vi "User Event Print.vi"(7 "Options":T1, 8 "error in (no error)":errorcluster, 9 "add EOL? (T)":bool=TRUE, 11 "String to Print":string) -> (0 "error out":errorcluster, 3 "Print":refnum<user-event>)   [LabVIEW 2018]
uses:
  Print Options.ctl
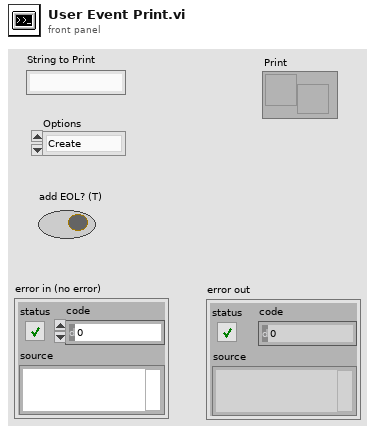
[diagram p1: front panel]
types:
  T1 = typedef "Print Options.ctl" = enum16{"Create", "Get Reference", "Print", "Print Header", "Close"}
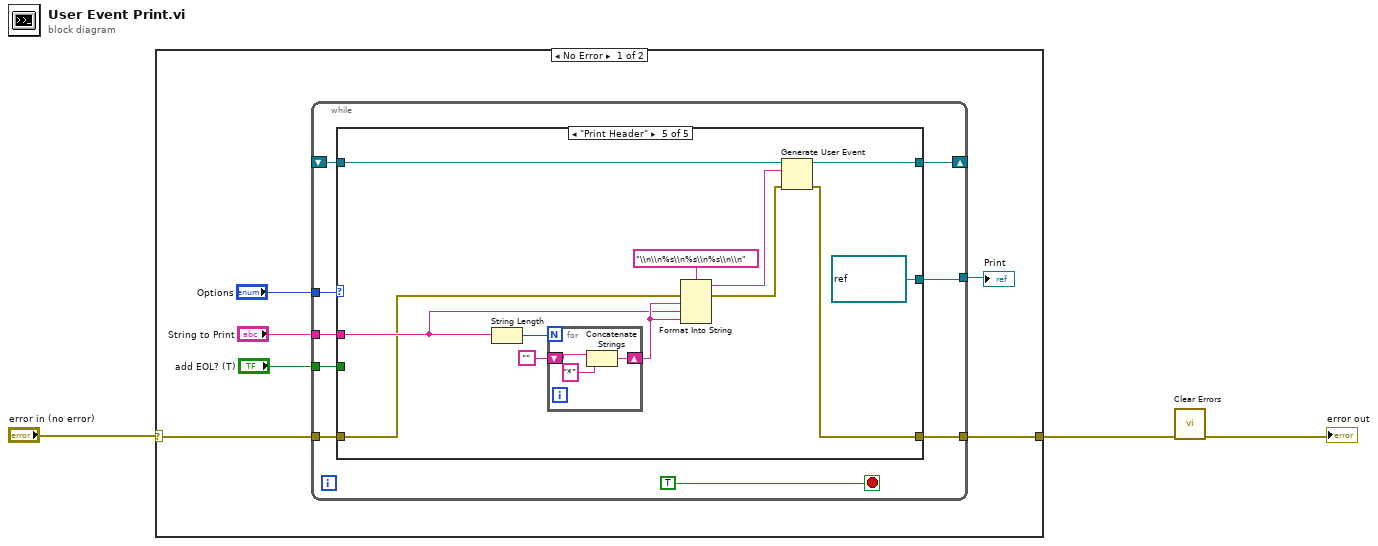
[diagram p0: block diagram]
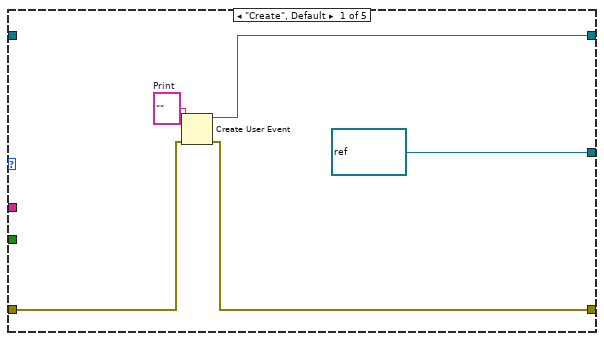
[diagram p2: hidden frame]
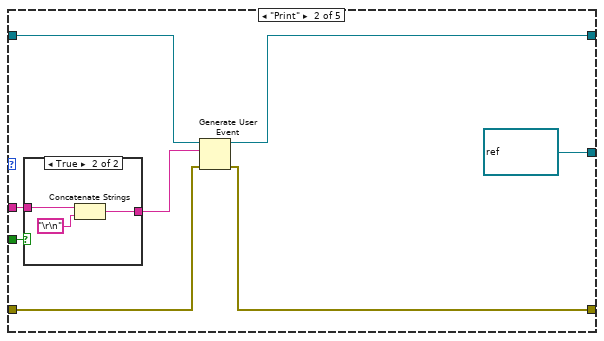
[diagram p3: hidden frame]
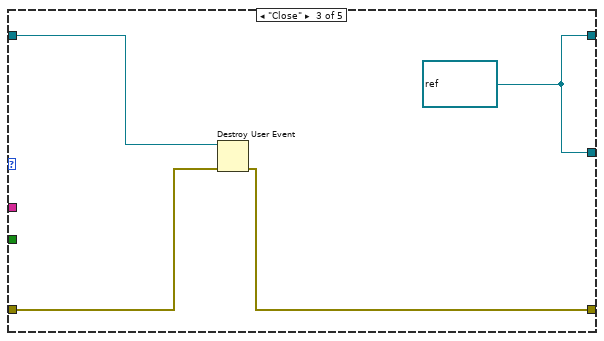
[diagram p5: hidden frame]
diagram:
  n1 = case shown="No Error" "error in (no error)" {
    selector: "error in (no error)" -> [w5 w57]
    tunnel: [w4 w57] -> w2
    frame No Error {
      n2 = while {
        tunnel: "Options" -> [w17]
        tunnel: "String to Print" -> [w16]
        tunnel: "add EOL? (T)" -> [w15]
        shift-right: [w14] -> _
        shift-left: _ -> [w13]
        tunnel: [w12] -> w6
        tunnel: w5 -> [w11]
        tunnel: [w10] -> w4
        stop <- TRUE stop-if-true
        n3 = case shown="\"Print Header\"" w17 {
          tunnel: w16 -> [_ w31 _ _ w45]
          tunnel: w15 -> [_ w29 _ _ _]
          tunnel: [w22 w27 w38 w41 w47] -> w14
          tunnel: w13 -> [_ w28 w39 w41 w53]
          tunnel: [refnum<user-event> refnum ("Print") refnum<user-event> refnum ("Print") w38 w41 refnum<user-event> refnum ("Print")] -> w12
          tunnel: w11 -> [w20 w25 w37 w40 w44]
          tunnel: [w19 w24 w36 w40 w42] -> w10
          frame "Create", Default {
            w23 = ""  # Print
            n4 = Create User Event(user event datatype=w23, error in=w20) -> (user event=w22:refnum<user-event>, error out=w19:errorcluster)
          }
          frame "Print" {
            n5 = case shown="True" w29 {
              tunnel: w31 -> [w32 w35]
              tunnel: [w32 w34] -> w30
              frame False {
              }
              frame True {
                n6 = Concatenate Strings(w35, "\r\n") -> (w34:string)
              }
            }
            n7 = Generate User Event(user event=w28, event data cluster=w30, error in=w25) -> (user event out=w27:refnum<user-event>, error out=w24:errorcluster)  [unwired: 1 in]
          }
          frame "Close" {
            w38 = refnum<user-event> refnum ("Print")
            n8 = Destroy User Event(user event=w39, error in=w37) -> (error out=w36:errorcluster)
          }
          frame "Get Reference" {
          }
          frame "Print Header" {
            n9 = String Length(string=w45) -> (length=w51:i32)
            n10 = for {
              N: w51 -> [_]
              shift-right: [w54] -> w49
              shift-left: "" -> [w55]
              n11 = Concatenate Strings(w55, "*") -> (w54:string)
            }
            n12 = Format Into String(format string="\\n\\n%s\\n%s\\n%s\\n\\n", error in=w44, w49, w45, w49) -> (resulting string=w46:string, error out=w43:errorcluster)  [unwired: 1 in]
            n13 = Generate User Event(user event=w53, event data cluster=w46, error in=w43) -> (user event out=w47:refnum<user-event>, error out=w42:errorcluster)  [unwired: 1 in]
          }
        }
      }
      "Print" <- w6
    }
    frame Error {
    }
  }
  n14 = call <vilib>:"Clear Errors.vi"("error in (no error)"=w2) -> ("error out"=→"error out":errorcluster)  [unwired: 5 in, 1 out]
